vi "Main.vi"(8 "error in":errorcluster, 11 "PythonConverter_GUI in":refnum<class "PythonConverter_GUI.lvclass">) -> (0 "error out":errorcluster, 3 "PythonConverter_GUI out":refnum<class "PythonConverter_GUI.lvclass">, 4 "main":string)   [LabVIEW 2014, in "PythonConverter_GUI.lvclass"]
uses:
  PythonConverter_GUI.lvclass
  <vilib>/Utility/error.llb/whitespace.ctl
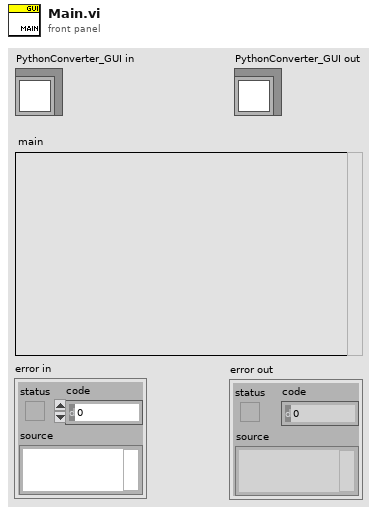
[diagram p1: front panel]
types:
  T1 = typedef "whitespace.ctl" = u16
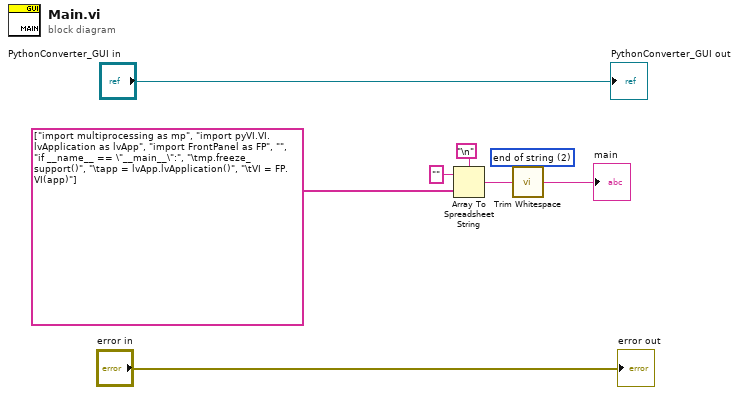
[diagram p0: block diagram]
diagram:
  w4 = T1 2 items=["both", "start of string", "end of string"] ("location (both)")
  n1 = Array To Spreadsheet String(delimiter (Tab)="\n", array=string[] ["import multiprocessing as mp", "import pyVI.VI.lvApplication as lvApp", "import FrontPanel as FP", "", "if __name__ == \"__main__\":", "\tmp.freeze_support()", "\tapp = lvApp.lvApplication()", "\tVI = FP.VI(app)"] ("parameters"), 3:"" ("format string")) -> (spreadsheet string=w5:string)
  n2 = call <vilib>:"Trim Whitespace.vi"("string"=w5, "location (both)"=w4) -> ("trimmed string"=→"main":string)
  "error out" <- "error in"
  "PythonConverter_GUI out" <- "PythonConverter_GUI in"
